vi "xw_correction_global_m.vi"() -> ()   [LabVIEW 2010]
panel:
  in  "ce":dbl format="%.2f"
  in  "cd":dbl format="%.2f"
  in  "cc":dbl format="%.2f"
  in  "cb":dbl format="%.2f"
  in  "ca":dbl format="%.2f"
  in  "c":dbl format="%.2f"
  in  "s2":dbl=0.7071067811865475 format="%.2f"
  in  "s1":dbl=0.7071067811865475 format="%.2f"
  in  "c2":dbl=0.7071067811865476 format="%.2f"
  in  "c1":dbl=0.7071067811865476 format="%.2f"
  in  "J1":dbl=1.0 format="%.5f"
  in  "alpha2":dbl=0.7853981633974483 format="%.2f"
  in  "alpha1":dbl=0.7853981633974483 format="%.2f"
  in  "rho":dbl=0.3 format="%.2f"
  in  "w'/U":dbl=0.16 format="%.2f"
  in  "v'/U":dbl=0.16 format="%.2f"
  in  "u'/U":dbl=0.2 format="%.2f"
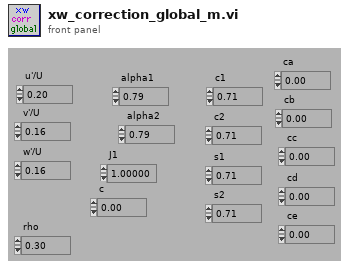
[diagram p1: front panel]
diagram:
